vi "ukol3.vi"() -> ()   [LabVIEW 2023]
uses:
  <vilib>/measure/maspectr.llb/FFT Spectrum (Mag-Phase) for 1 Chan.vi
  <vilib>/addons/Time Frequency Analysis/Transform.llb/TFA STFT (Waveform).vi
  <vilib>/measure/NI_MAPro.lvlib
  <vilib>/addons/_Advanced Signal Processing/NI_AdvSigProcTFA.lvlib
panel:
  out "Waveform Graph 2":waveform(dbl)(graph)
  in  "stop":bool
  in  "Noise STD":dbl format="%.2p"
  out "Coefficients":dbl[][](graph)
  out "Waveform Graph":cluster{"f0":dbl, "df":dbl, "magnitude":dbl[]}(graph)
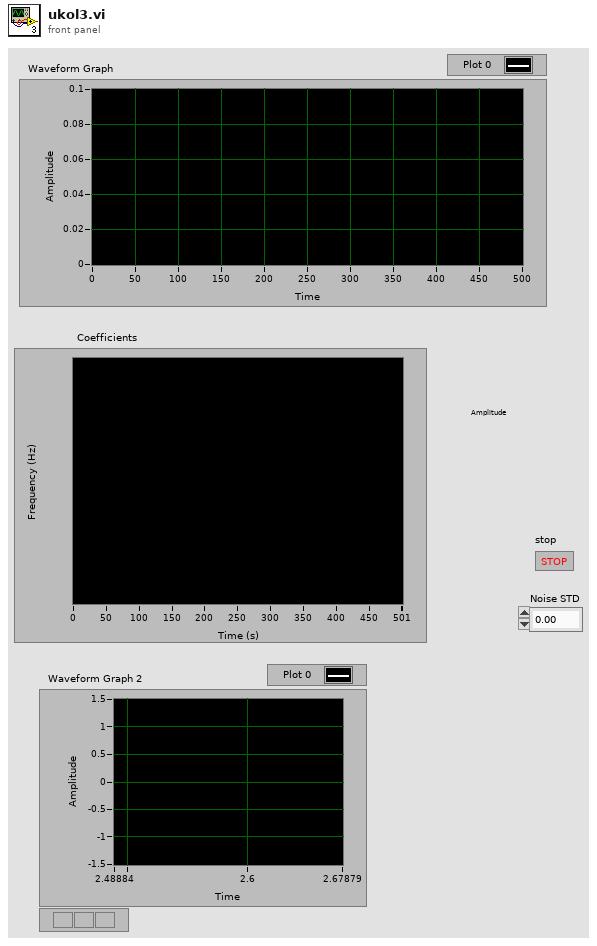
[diagram p1: front panel]
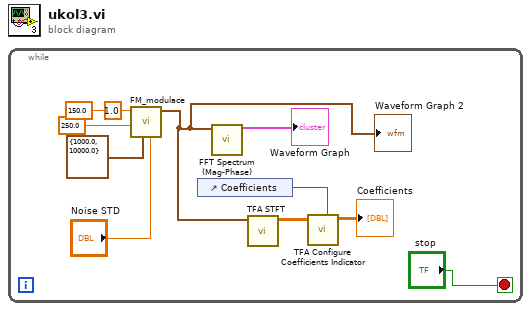
[diagram p0: block diagram]
diagram:
  n1 = while {
    stop <- "stop" stop-if-true
    n2 = call "FM_modulace.vi"("Noise STD"="Noise STD", "Sampling info"=cluster{"Fs":dbl, "#s":dbl} {"Fs"=1000.0, "#s"=10000.0}, "Nosna Frekvence (Hz)"=250.0, "Frekvencni zdvih (Hz)"=150.0, "Modulacni Frekvence (Hz)"=1.0) -> ("Modulovany signal"=w1:waveform(dbl))  [unwired: 3 in, 3 out]
    "Waveform Graph 2" <- w1
    n3 = control-ref of="Coefficients"() -> (w9:refnum<vi>)
    n4 = call-poly <vilib>:"FFT Spectrum (Mag-Phase).vi"("time signal"=w1) -> ("magnitude"=→"Waveform Graph":cluster{"f0":dbl, "df":dbl, "magnitude":dbl[]})  [unwired: 6 in, 4 out]
    n5 = call-poly <vilib>:"TFA STFT.vi"("signal"=w1) -> ("STFT coef"=w7:cdb[][])  [unwired: 8 in, 2 out]
    n6 = call <vilib>:"TFA Configure Coefficients Indicator.vi"("reference of TF coefficients indicator"=w9, "TF coefficients"=w7) -> ("TF coefficients indicator"=→"Coefficients":dbl[][])  [unwired: 5 in, 4 out]
  }
